vi "Test Get Registered Path.vi"() -> ()   [LabVIEW 2021, in "Path Utilities.lvlib"]
uses:
  Path Utilities.lvlib
panel:
  out "Cleared Paths":path[](array[path])
  out "Result":bool
  in  "Tab Control":enum32{"1", "2", "3", "4"}(tab)
  out "Test 1":T1
  out "Test 2":T1
  out "Test 3":T1
  out "Test 4":T1
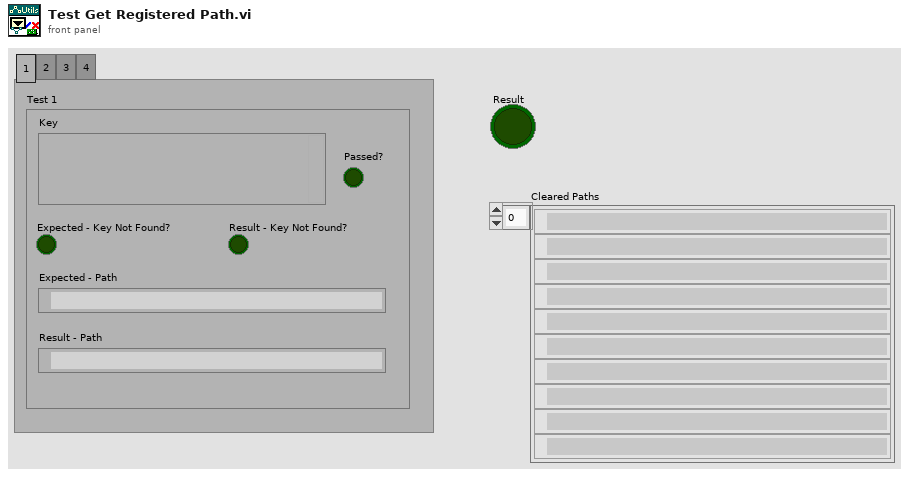
[diagram p1: front panel]
types:
  T1 = cluster{"Key":variant, "Expected - Key Not Found?":bool, "Result - Key Not Found?":bool, "Expected - Path":path, "Result - Path":path, "Passed?":bool}
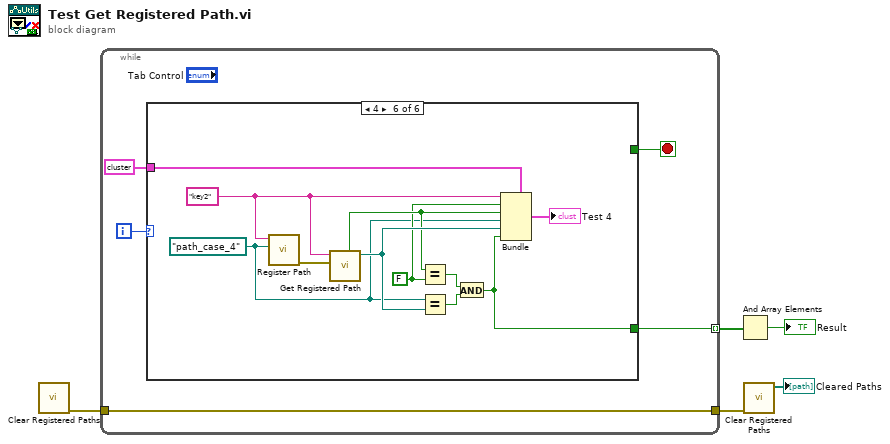
[diagram p0: block diagram]
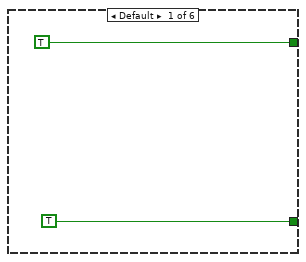
[diagram p2: hidden frame]
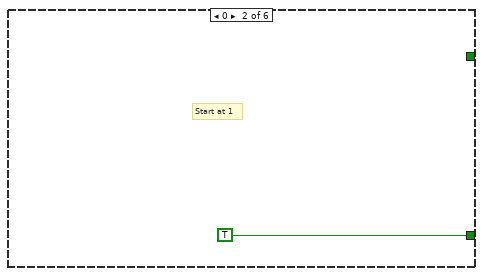
[diagram p3: hidden frame]
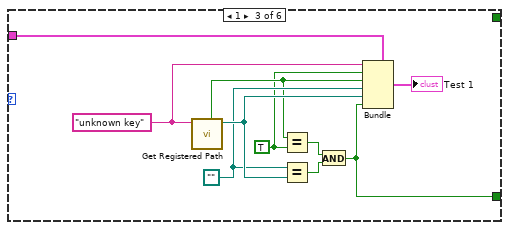
[diagram p4: hidden frame]
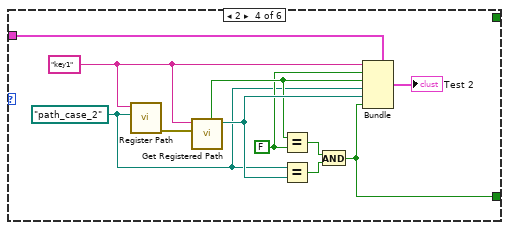
[diagram p5: hidden frame]
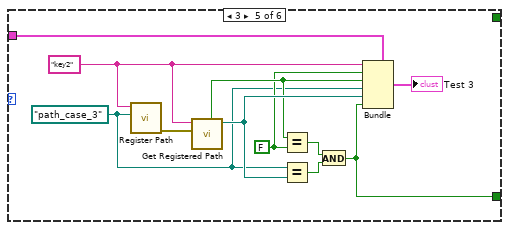
[diagram p6: hidden frame]
diagram:
  n1 = call "Clear Registered Paths.vi"() -> ("error out"=w5:errorcluster)  [unwired: 10 in, 1 out]
  n2 = while {
    tunnel: [w8] -> w1 mode=indexing
    tunnel: w5 -> [w7]
    tunnel: [w7] -> w2
    i -> [w10]
    stop <- w9 stop-if-true
    n3 = case shown="4" w10 {
      tunnel: [TRUE _ _ _ _ _] -> w9
      tunnel: [TRUE TRUE w15 w27 w38 w49] -> w8
      tunnel: T1 {"Key"=variant, "Expected - Key Not Found?"=FALSE, "Result - Key Not Found?"=FALSE, "Expected - Path"=path "", "Result - Path"=path "", "Passed?"=FALSE} ("Test 1") -> [_ _ w23 w34 w45 w56]
      frame Default {
      }
      frame 0 {
        # "Start at 1"
      }
      frame 1 {
        w14 = "unknown key"
        w18 = TRUE ("y")
        w20 = path ""
        n4 = call "Get Registered Path.vi"("Key"=w14) -> ("Registered Path"=w21:path, "Key Not Found?"=w19:bool)  [unwired: 8 in, 1 out]
        n5 = Equal?(x=w19, y=w18) -> (x = y?=w16:bool)
        n6 = Equal?(x=w20, y=w21) -> (x = y?=w17:bool)
        n7 = And(x=w16, y=w17) -> (x .and. y?=w15:bool)
        n8 = Bundle(cluster=w23, "Key"=w14, "Expected - Key Not Found?"=w18, "Result - Key Not Found?"=w19, "Expected - Path"=w20, "Result - Path"=w21, "Passed?"=w15) -> (→"Test 1":T1)
      }
      frame 2 {
        w24 = path "path_case_2" ("Path")
        w25 = "key1"
        w30 = FALSE ("y")
        n9 = call "Register Path.vi"("Path"=w24, "Key"=w25) -> ("error out"=w26:errorcluster)  [unwired: 7 in, 2 out]
        n10 = call "Get Registered Path.vi"("error in (no error)"=w26, "Key"=w25) -> ("Registered Path"=w32:path, "Key Not Found?"=w31:bool)  [unwired: 7 in, 1 out]
        n11 = Equal?(x=w31, y=w30) -> (x = y?=w28:bool)
        n12 = Equal?(x=w24, y=w32) -> (x = y?=w29:bool)
        n13 = And(x=w28, y=w29) -> (x .and. y?=w27:bool)
        n14 = Bundle(cluster=w34, "Key"=w25, "Expected - Key Not Found?"=w30, "Result - Key Not Found?"=w31, "Expected - Path"=w24, "Result - Path"=w32, "Passed?"=w27) -> (→"Test 2":T1)
      }
      frame 3 {
        w35 = path "path_case_3" ("Path")
        w36 = "key2"
        w41 = FALSE ("y")
        n15 = call "Register Path.vi"("Path"=w35, "Key"=w36) -> ("error out"=w37:errorcluster)  [unwired: 7 in, 2 out]
        n16 = call "Get Registered Path.vi"("error in (no error)"=w37, "Key"=w36) -> ("Registered Path"=w43:path, "Key Not Found?"=w42:bool)  [unwired: 7 in, 1 out]
        n17 = Equal?(x=w42, y=w41) -> (x = y?=w39:bool)
        n18 = Equal?(x=w35, y=w43) -> (x = y?=w40:bool)
        n19 = And(x=w39, y=w40) -> (x .and. y?=w38:bool)
        n20 = Bundle(cluster=w45, "Key"=w36, "Expected - Key Not Found?"=w41, "Result - Key Not Found?"=w42, "Expected - Path"=w35, "Result - Path"=w43, "Passed?"=w38) -> (→"Test 3":T1)
      }
      frame 4 {
        w46 = path "path_case_4" ("Path")
        w47 = "key2"
        w52 = FALSE ("y")
        n21 = call "Register Path.vi"("Path"=w46, "Key"=w47) -> ("error out"=w48:errorcluster)  [unwired: 7 in, 2 out]
        n22 = call "Get Registered Path.vi"("error in (no error)"=w48, "Key"=w47) -> ("Registered Path"=w54:path, "Key Not Found?"=w53:bool)  [unwired: 7 in, 1 out]
        n23 = Equal?(x=w53, y=w52) -> (x = y?=w50:bool)
        n24 = Equal?(x=w46, y=w54) -> (x = y?=w51:bool)
        n25 = And(x=w50, y=w51) -> (x .and. y?=w49:bool)
        n26 = Bundle(cluster=w56, "Key"=w47, "Expected - Key Not Found?"=w52, "Result - Key Not Found?"=w53, "Expected - Path"=w46, "Result - Path"=w54, "Passed?"=w49) -> (→"Test 4":T1)
      }
    }
  }
  n27 = And Array Elements(Boolean array=w1) -> (logical AND=→"Result":bool)
  n28 = call "Clear Registered Paths.vi"("error in (no error)"=w2) -> ("Cleared Paths"=→"Cleared Paths":path[])  [unwired: 9 in, 1 out]
